vi "NicmosGetReadout.vi"(9 "error in (no error)":errorcluster caption="error out (no error)") -> (0 "READOUT out":T1, 6 "error out":errorcluster)   [LabVIEW 2009]
uses:
  Controls/NICMOS.READOUT.ctl
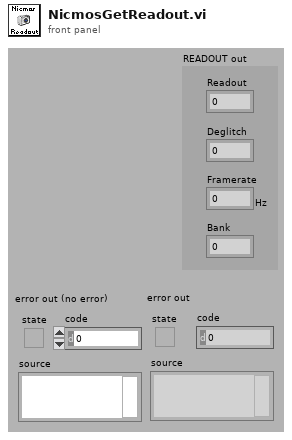
[diagram p1: front panel]
types:
  T1 = typedef "NICMOS.READOUT.ctl" = cluster{"Readout":i32, "Deglitch":i32, "Framerate":dbl[unit], "Bank":i32}
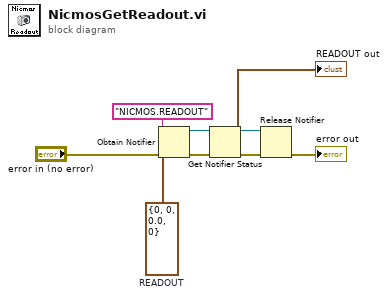
[diagram p0: block diagram]
diagram:
  w8 = T1 {"Readout"=0, "Deglitch"=0, "Framerate"=0.0, "Bank"=0}  # READOUT
  n1 = Obtain Notifier(name (unnamed)="NICMOS.READOUT" ("nom (aucun)"), notification data type=w8, error in (no error)="error in (no error)") -> (notifier out=w1:refnum<notifier>, error out=w2:errorcluster)  [unwired: 1 in, 1 out]
  n2 = Get Notifier Status(notifier=w1, error in (no error)=w2) -> (notifier out=w4:refnum<notifier>, current notification=→"READOUT out":T1, error out=w6:errorcluster)  [unwired: 2 out]
  n3 = Release Notifier(notifier=w4, error in (no error)=w6) -> (error out=→"error out":errorcluster)  [unwired: 1 in, 2 out]
